vi "Constants.vi"() -> ()   [LabVIEW 2014]
panel:
  in  "InferredZPositionClamp":sgl
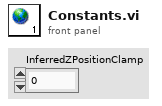
[diagram p1: front panel]
diagram:
